vi "Get Session.vi"(11 "XNET Base CFG in":refnum<class "XNET Base CFG.lvclass">) -> (2 "Session":refnum<k21>, 3 "XNET Base CFG out":refnum<class "XNET Base CFG.lvclass">)   [LabVIEW 2024, in "XNET Base CFG.lvclass"]
uses:
  XNET Base CFG.lvclass
  XNET Base CFG.lvclass/XNET Base CFG.ctl
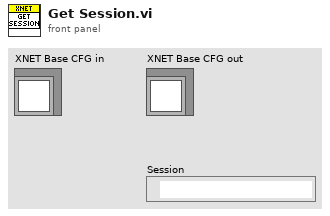
[diagram p1: front panel]
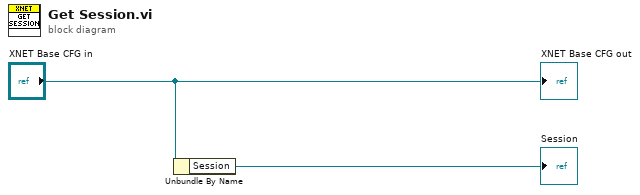
[diagram p0: block diagram]
diagram:
  n1 = Unbundle By Name("XNET Base CFG in") -> ("Session"=→"Session":refnum<k21>)
  "XNET Base CFG out" <- "XNET Base CFG in"
